vi "SVPO Envelope Detection (1 Ch DBL WDT).vi"(0 "scaled signal [EU]":waveform(dbl)={"t0"=timestamp(0 s since 1904-01-01), "dt"=0.0, "Y"=[]}, 1 "reset? (F)":bool, 9 "band specification":T1={"center frequency [Hz]"=4800.0, "span [Hz]"=2000.0}) -> (4 "envelope signal [EU]":waveform(dbl))   [LabVIEW 2017, in "SoundVib_FaultAnalysis.lvlib"]
doc: "Extracts the modulating signal, or envelope signal, from an amplitude-modulated signal. You can use the envelope detection technique to identify the mechanical faults that have amplitude-modulating effect on the vibration signal of a machine. Use this VI on embedded targets that have limited computational resources. Wire data to the <B>scaled signal [EU]</B> input to determine the polymorphic instance to use or manually select the instance."
uses:
  <vilib>/addons/Sound and Vibration/Order Analysis/Fault Analysis/SoundVib_FaultAnalysis.lvlib
  <vilib>/addons/Sound and Vibration/Order Analysis/Fault Analysis/SubVIs/sv_Shift and Low Pass Filter (1 Channel) with IC.vi
  <vilib>/addons/Sound and Vibration/Order Analysis/Resample Order Tracking/SubVIs/oa_Calculate CIC Decimation Filter Coefficients.vi
  <vilib>/addons/Sound and Vibration/Order Analysis/Fault Analysis/SubVIs/sv_Compute Shift and Low Pass Filter with IC.vi
  <vilib>/addons/Sound and Vibration/Order Analysis/Resample Order Tracking/SubVIs/OAT Frequency Shift (Mixer).vi
  <vilib>/addons/Sound and Vibration/Order Analysis/Resample Order Tracking/SubVIs/oa_Decimation with CIC and Compensation Filter.vi
  <vilib>/addons/Sound and Vibration/Order Analysis/Fault Analysis/SubVIs/oa_Demodulation Initial States (1 Channel).vi
  <vilib>/addons/Sound and Vibration/Order Analysis/Adv Resampling/OAT Single Stage Decimation with IC.vi
  <vilib>/addons/Sound and Vibration/Order Analysis/Resample Order Tracking/SubVIs/OAT CIC Decimation.vi
  <vilib>/addons/Sound and Vibration/Order Analysis/Resample Order Tracking/SubVIs/oa_Interpolate Zeros Between Samples.vi
  <vilib>/addons/Sound and Vibration/Order Analysis/Resample Order Tracking/SubVIs/oa_Calculate Delay of CIC Decimation Interpolation Filter.vi
  <vilib>/addons/Sound and Vibration/Order Analysis/Resample Order Tracking/SubVIs/oa_Create CIC Compensation Filter.vi
  <vilib>/addons/Sound and Vibration/Order Analysis/Resample Order Tracking/SubVIs/oa_Create CIC LP Truncation Filter.vi
  <vilib>/addons/Sound and Vibration/Order Analysis/Fault Analysis/SubVIs/oa_Calculate Decimation Factor and New Fs.vi
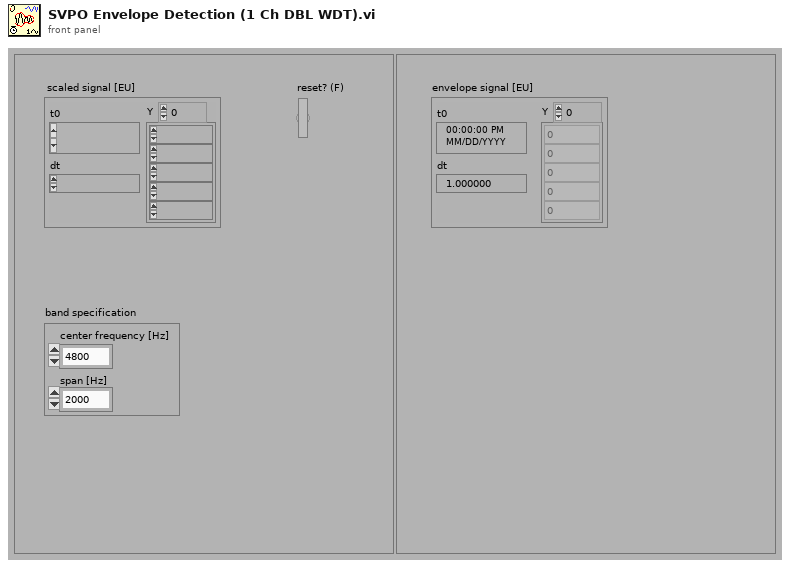
[diagram p1: front panel]
types:
  T1 = cluster{"center frequency [Hz]":dbl, "span [Hz]":dbl}
  T2 = typedef "svc_Envelope Detection State.ctl" = cluster{"filter settings":cluster{"CIC Settings":cluster{"Numeric":i32, i32, i32}, "filters":T3[], "delay":i32, "interpolation factor":i32}, "filter state":cluster{"t0":dbl, "phase":dbl, "real filter state":cluster{cluster{dbl[]}, cluster{dbl[]}[]}, "imaginary filter state":cluster{cluster{dbl[]}, cluster{dbl[]}[]}, "delay":i32}, "reset pending":bool}
  T3 = typedef "OAT Decimation Filter.ctl" = cluster{"coefficients":dbl[], "factor":i32}
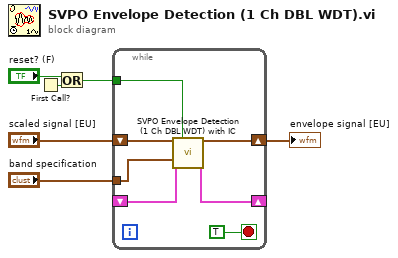
[diagram p0: block diagram]
diagram:
  n1 = First Call?() -> (First Call?: T/F=w5:bool)
  n2 = Or(x="reset? (F)", y=w5) -> (x .or. y?=w4:bool)
  n3 = while {
    tunnel: w4 -> [w13]
    tunnel: "band specification" -> [w10]
    shift-right: [w9] -> _
    shift-left: _ -> [w8]
    shift-right: [w11] -> w2
    shift-left: "scaled signal [EU]" -> [w12]
    stop <- TRUE stop-if-true
    n4 = call <vilib>:"SVPO Envelope Detection (1 Ch DBL WDT) with IC.vi"("scaled signal [EU]"=w12, "reset? (F)"=w13, "band specification"=w10, "initial conditions"=w8) -> ("envelope signal [EU]"=w11:waveform(dbl), "final conditions"=w9:T2)  [unwired: 10 in]
  }
  "envelope signal [EU]" <- w2
